vi "Calculate_NXY_Coords_and_Dim_Info_of_Selected_Coreset_Indices.vi"(8 "error in (no error)":errorcluster, 10 "Selected_Feature_Coords":T1[](array[typedef]), 11 "NNPC_Instance":T4={"Name"="", "NN"={"Name"="wrn", "No of Layers"=0, "mBatch"=1, "Layers"=[], "Dimty"=enum."In3D_Out3D", "Dims_In"={"C"=-1, "H"=-1, "W"=-1}, "Dims_Out"={"C"=-1, "H"=-1, "W"=-1}, "Working_Dir"=path "", "Train?"=FALSE, "Train_Params"={"Optimizer"=enum."SGD", "Beta_1"=0.999, "Beta_2"=0.999, "Weight Decay(L1)"=0.0, "Weight Decay(L2)"=0.0, "Data_Sampling"=enum."Random"}, "LR_Update_Policy"={"Policy_Type"=enum."Manual", "LR0"=0.0, "k"=0.0, "WarmUp_Policy"=enum."Step", "WarmUp_Iter"=100, "WarmUp_Ratio"=10.0}, "Session Data"={"Epochs"=0.0, "Tot_Iter"=1, "LR"=0.0, "LR_iter"=1}, "Ground_truth"={"Y"=variant}, "NNg_hdls"={"cudnn"=2143106709504, "cublas"=2177817002560, "stream"=2141212075440, "curand"=2143055681792}, "NN_Device"=enum."GPU", "GPU Id"=0, "Labels"=[], "Loss_Type"=enum."MSE", "Loss_Cfg_Prms"=variant, "NNG_WS"={"NNG_WS_Mem"=refnum, "Max_WS_Size"=-1}, "DryRun?"=FALSE}, "MemBank_Data"={"MemBank"=variant, "MemBank Norm"=variant}} {"NN"."LR_Update_Policy"."WarmUp_Ratio" min=1; "NN"."LR_Update_Policy"."WarmUp_Iter" min=1; "NN"."LR_Update_Policy"."LR0" format="%.7f"}) -> (0 "error out":errorcluster, 3 "Selected_Coreset_Element_Info":T2)   [LabVIEW 2020]
uses:
  <vilib>/Ngene/DeepLTK Anomaly Detection Addon/Toolkit/API/Controls/NNPC_Instance.ctl
  <vilib>/Ngene/Deep Learning Toolkit/Toolkit/NN_Network/Controls/NN.ctl
  <vilib>/Ngene/Deep Learning Toolkit/Toolkit/NN_Layers/Controls/NN_Layer_ref.ctl
  <vilib>/Ngene/Deep Learning Toolkit/Toolkit/NN_Network/Controls/NN_In_Out_Dim-ty.ctl
  <vilib>/Ngene/Deep Learning Toolkit/Toolkit/NN_Data/API/NN_Dims(C,H,W).ctl
  <vilib>/Ngene/Deep Learning Toolkit/Toolkit/NN_Train/Controls/NN_Train_Params.ctl
  <vilib>/Ngene/Deep Learning Toolkit/Toolkit/NN_Train/Controls/NN_Train_Optimizer.ctl
  <vilib>/Ngene/Deep Learning Toolkit/Toolkit/NN_Train/Controls/NN_Train_Data_Sampling.ctl
  <vilib>/Ngene/Deep Learning Toolkit/Toolkit/NN_Train/Controls/NN_LR_Policy_Cfg.ctl
  <vilib>/Ngene/Deep Learning Toolkit/Toolkit/NN_Train/Controls/NN_LR_Policy_Type.ctl
  <vilib>/Ngene/Deep Learning Toolkit/Toolkit/NN_Train/Controls/NN_Train_Session_Data.ctl
  <vilib>/Ngene/Deep Learning Toolkit/Toolkit/NN_Data/Controls/NN_Ground_truth.ctl
  <vilib>/Ngene/Deep Learning Toolkit/Toolkit/NNg/cuda/Controls/nng_cuda_handles.ctl
  <vilib>/Ngene/Deep Learning Toolkit/Toolkit/NN_Network/Controls/NN_Device.ctl
  <vilib>/Ngene/Deep Learning Toolkit/Toolkit/NN_Train/Controls/NN_Loss_Type.ctl
  <vilib>/Ngene/Deep Learning Toolkit/Toolkit/NNg/Network/WS/Controls/NNG_WS.ctl
  <vilib>/Ngene/Deep Learning Toolkit/Toolkit/NNg/Network/WS/Controls/NNg_WS_Mem_DVR.ctl
  <vilib>/Ngene/Deep Learning Toolkit/Toolkit/NNg/cuda/Controls/cuda_Mem_desc.ctl
  <vilib>/Ngene/DeepLTK Anomaly Detection Addon/Toolkit/API/Controls/MemBank_and_Norm_Variants.ctl
  Controls/Selected_Coreset_Elements_and_Dim_Stride_Info.ctl
  Controls/Dims(2D)ctl.ctl
  <vilib>/Ngene/DeepLTK Anomaly Detection Addon/Toolkit/API/Controls/Feature_Coords(Idx,i,j).ctl
  <vilib>/Ngene/Deep Learning Toolkit/Toolkit/Deep_Learning_Toolkit_by_Ngene.lvlib
  <vilib>/Ngene/DeepLTK Anomaly Detection Addon/Toolkit/DeepLTK_Anomaly_Detection_Addon.lvlib
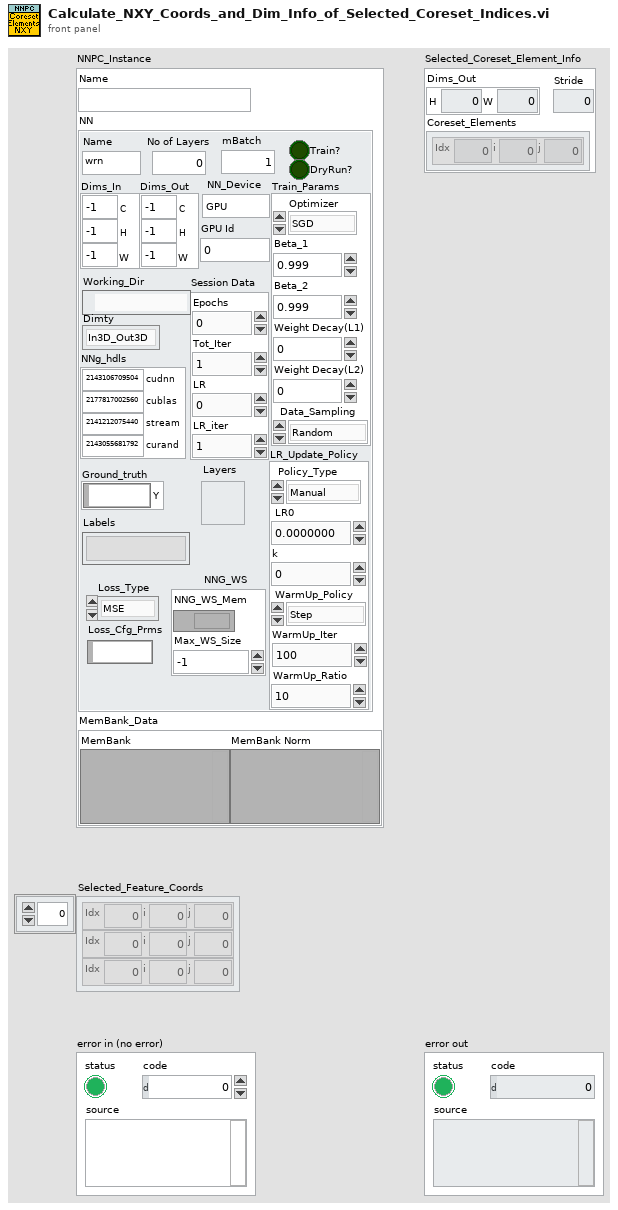
[diagram p1: front panel]
types:
  T1 = typedef "DeepLTK_Anomaly_Detection_Addon.lvlib/Feature_Coords(Idx,i,j).ctl" = cluster{"Idx":i32, "i":i32, "j":i32}
  T2 = typedef "Selected_Coreset_Elements_and_Dim_Stride_Info.ctl" = cluster{"Dims_Out":T3, "Stride":i32, "Coreset_Elements":T1[]}
  T3 = typedef "Dims(2D)ctl.ctl" = cluster{"H":i32, "W":i32}
  T4 = typedef "DeepLTK_Anomaly_Detection_Addon.lvlib/NNPC_Instance.ctl" = cluster{"Name":string, "NN":T5, "MemBank_Data":T21}
  T5 = typedef "Deep_Learning_Toolkit_by_Ngene.lvlib/NN.ctl" = cluster{"Name":string, "No of Layers":i32, "mBatch":i32, "Layers":T6[], "Dimty":T7, "Dims_In":T8, "Dims_Out":T8, "Working_Dir":path, "Train?":bool, "Train_Params":T9, "LR_Update_Policy":T12, "Session Data":T14, "Ground_truth":T15, "NNg_hdls":T16, "NN_Device":T17, "GPU Id":i32, "Labels":string[], "Loss_Type":T18, "Loss_Cfg_Prms":variant, "NNG_WS":T19, "DryRun?":bool}
  T6 = typedef "Deep_Learning_Toolkit_by_Ngene.lvlib/NN_Layer_ref.ctl" = refnum<file>
  T7 = typedef "Deep_Learning_Toolkit_by_Ngene.lvlib/NN_In_Out_Dim-ty.ctl" = enum8{"In1D_Out1D", "In3D_Out1D", "In3D_Out3D", "In3D_OutBBox"}
  T8 = typedef "Deep_Learning_Toolkit_by_Ngene.lvlib/NN_Dims(C,H,W).ctl" = cluster{"C":i32, "H":i32, "W":i32}
  T9 = typedef "Deep_Learning_Toolkit_by_Ngene.lvlib/NN_Train_Params.ctl" = cluster{"Optimizer":T10, "Beta_1":sgl, "Beta_2":sgl, "Weight Decay(L1)":sgl, "Weight Decay(L2)":sgl, "Data_Sampling":T11}
  T10 = typedef "Deep_Learning_Toolkit_by_Ngene.lvlib/NN_Train_Optimizer.ctl" = enum16{"SGD", "Adam", "Adagrad", "Adadelta", "RMSProp", "Nesterov"}
  T11 = typedef "Deep_Learning_Toolkit_by_Ngene.lvlib/NN_Train_Data_Sampling.ctl" = enum16{"Random", "Sequential"}
  T12 = typedef "Deep_Learning_Toolkit_by_Ngene.lvlib/NN_LR_Policy_Cfg.ctl" = cluster{"Policy_Type":T13, "LR0":dbl, "k":sgl, "WarmUp_Policy":enum16{"Step", "Ramp"}, "WarmUp_Iter":i32, "WarmUp_Ratio":sgl}
  T13 = typedef "Deep_Learning_Toolkit_by_Ngene.lvlib/NN_LR_Policy_Type.ctl" = enum16{"Manual", "Step", "Exp", "1/t"}
  T14 = typedef "Deep_Learning_Toolkit_by_Ngene.lvlib/NN_Train_Session_Data.ctl" = cluster{"Epochs":sgl, "Tot_Iter":i32, "LR":sgl, "LR_iter":i32}
  T15 = typedef "Deep_Learning_Toolkit_by_Ngene.lvlib/NN_Ground_truth.ctl" = cluster{"Y":variant}
  T16 = typedef "Deep_Learning_Toolkit_by_Ngene.lvlib/nng_cuda_handles.ctl" = cluster{"cudnn":u64, "cublas":u64, "stream":u64, "curand":u64}
  T17 = typedef "Deep_Learning_Toolkit_by_Ngene.lvlib/NN_Device.ctl" = enum16{"CPU", "GPU"}
  T18 = typedef "Deep_Learning_Toolkit_by_Ngene.lvlib/NN_Loss_Type.ctl" = enum16{"None", "MSE", "CrossEntropy", "YOLO_v2", "YOLO_v4"}
  T19 = typedef "Deep_Learning_Toolkit_by_Ngene.lvlib/NNG_WS.ctl" = cluster{"NNG_WS_Mem":T20, "Max_WS_Size":i64}
  T20 = typedef "Deep_Learning_Toolkit_by_Ngene.lvlib/NNg_WS_Mem_DVR.ctl" = refnum<data-value>
  T21 = typedef "DeepLTK_Anomaly_Detection_Addon.lvlib/MemBank_and_Norm_Variants.ctl" = cluster{"MemBank":variant, "MemBank Norm":variant}
  T22 = typedef "Deep_Learning_Toolkit_by_Ngene.lvlib/NN_Layer.ctl" = cluster{"Name":string, "Layer_Data":T23, "Layer_Type":T24, "Dims_In":T8, "Layers_In":T6[], "Dims_Out":T8, "Layers_Out":T6[], "Metrics":T25, "GPU_Data":T26, "mBatch":i32, "NN_Device":T17, "NNg_hdls":T16, "Train?":bool, "Dimty":T27, "RecptField":T28, "Idx":i32}
  T23 = typedef "Deep_Learning_Toolkit_by_Ngene.lvlib/NN_Layer_Data_Refnum.ctl" = refnum<file>
  T24 = typedef "Deep_Learning_Toolkit_by_Ngene.lvlib/NN_Layer_Type.ctl" = enum16{"Input1D", "Input3D", "Conv1D", "Conv2D", "Conv2D_Adv", "MaxPool", "AvgPool", "UpSample", "DropOut3D", "ShortCut", "Concat", "SoftMax3D", "FC", "DropOut", "Softmax", "Flatten", "YOLO_v2", "YOLO_v4", "Activation", "BatchNormalization", "LayerNormalization", "Scale", "Unsupported"}
  T25 = typedef "Deep_Learning_Toolkit_by_Ngene.lvlib/NN_Layer_Metrics.ctl" = cluster{"Data":dbl, "Params":dbl, "Ops":dbl}
  T26 = typedef "Deep_Learning_Toolkit_by_Ngene.lvlib/NNg_Layer_Data_Refnum.ctl" = refnum<file>
  T27 = typedef "Deep_Learning_Toolkit_by_Ngene.lvlib/NN_Layer_Dimty.ctl" = enum16{"1D", "3D"}
  T28 = typedef "Deep_Learning_Toolkit_by_Ngene.lvlib/NN_Layer_RF_State.ctl" = cluster{"Dims":T29, "J":T29}
  T29 = typedef "Deep_Learning_Toolkit_by_Ngene.lvlib/NN_Dims(V,H).ctl" = cluster{"V":i32, "H":i32}
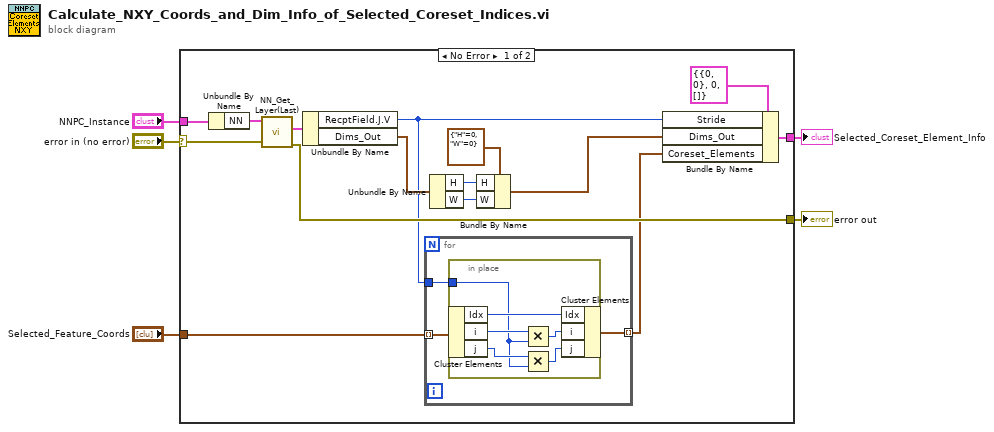
[diagram p0: block diagram]
diagram:
  n1 = case shown="No Error" "error in (no error)" {
    selector: "error in (no error)" -> [w20 w30]
    tunnel: [w19 w30] -> w4
    tunnel: "NNPC_Instance" -> [w17 _]
    tunnel: [w12 _] -> w2
    tunnel: "Selected_Feature_Coords" -> [w8 _]
    frame No Error {
      n2 = Unbundle By Name(w17) -> ("NN"=w18:T5)
      n3 = call <vilib>:"NN_Get_Layer(Last).vi"("error in (no error)"=w20, "NN in"=w18) -> ("error out"=w19:errorcluster, "Last_Layer"=w13:T22)  [unwired: 6 in, 2 out]
      n4 = Unbundle By Name(w13) -> ("RecptField.J.V"=w10:i32, "Dims_Out"=w11:T8)
      n5 = for {
        tunnel: w10 -> [w22]
        tunnel: w8 -> [w23] mode=indexing
        tunnel: [w21] -> w7 mode=indexing
        n6 = in-place {
          in-place-border: w22 -> [w24]
          n7 = in-place-cluster #1(w23) -> ("Idx"=w29:i32, "i"=w28:i32, "j"=w27:i32)
          n8 = Multiply(x=w28, y=w24) -> (x*y=w25:i32)
          n9 = Multiply(x=w27, y=w24) -> (x*y=w26:i32)
          n10 = in-place-cluster #1("Idx"=w29, "i"=w25, "j"=w26) -> (w21:T1)
        }
      }
      n11 = Unbundle By Name(w11) -> ("H"=w15:i32, "W"=w14:i32)
      n12 = Bundle By Name(cluster=T3 {"H"=0, "W"=0} ("Dims(2D)"), "H"=w15, "W"=w14) -> (w6:T3)
      n13 = Bundle By Name(cluster=T2 {"Dims_Out"={"H"=0, "W"=0}, "Stride"=0, "Coreset_Elements"=[]} ("Selected_Coreset_Element_Info 2"), "Stride"=w10, "Dims_Out"=w6, "Coreset_Elements"=w7) -> (w12:T2)
    }
    frame Error {
    }
  }
  "error out" <- w4
  "Selected_Coreset_Element_Info" <- w2
